vi "comm playing sender.vi"() -> ()   [LabVIEW 2009]
uses:
  UDP Lib/UDP Network Location.ctl
  <vilib>/Platform/TimedLoop/XDataNode/XDataNode.xnode
  <vilib>/Platform/TimedLoop/XDataNode/loadlvalarms.vi
  <vilib>/Platform/TimedLoop/XDataNode/timing_clust.ctl
  <vilib>/Platform/TimedLoop/XDataNode/nitl_modes.ctl
  <vilib>/Platform/TimedLoop/XDataNode/wakeup.ctl
  <vilib>/Platform/TimedLoop/XDataNode/XDNodeRunTimeDep.lvlib
panel:
  out "Network Location":T1
  out "Receive Data":string
  in  "Read Timeout":i32=1000
  in  "Local Port":u16=8800
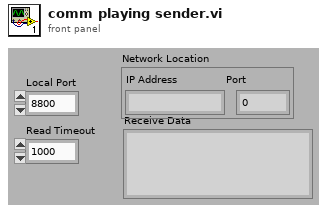
[diagram p1: front panel]
types:
  T1 = typedef "UDP Network Location.ctl" = cluster{"IP Address":string, "Port":u16}
  T2 = typedef "XDNodeRunTimeDep.lvlib/timing_clust.ctl" = cluster{"Expected End [f-1]":u64, "Actual End [f-1]":u64, "Finished Late? [f-1]":bool, "Expected End [i-1]":u64, "Actual End [i-1]":u64, "Finished Late? [i-1]":bool, "Expected Start [i]":u64, "Actual Start [i]":u64, "Expected Start [f]":u64, "Actual Start [f]":u64, "Source Name":string, "Structure Name":string, "Period":i64, "Deadline":i64, "Offset":i64, "Start":i64, "Priority":i32, "Timeout":i32, "Mode":T3, "Wakeup Reason":T4, "Error":errorcluster, "Source Type":string, "Secondary Source Type":string, "Global End Time":u64, "Global Start Time":u64, "Frame Duration":u64, "Iteration Duration":u64, "Assigned CPU":i32, "I/O Scan Engine Mode":u32}
  T3 = typedef "XDNodeRunTimeDep.lvlib/nitl_modes.ctl" = enum32{"No Change", "Process missed periods, maintain original phase", "Discard missed periods, maintain original phase", "Process missed periods, ignore original phase", "Discard missed periods, ignore original phase"}
  T4 = typedef "XDNodeRunTimeDep.lvlib/wakeup.ctl" = enum32{"Normal", "Aborted", "Asynchronous wakeup", "Timing source error", "Timed loop error", "Timeout"}
  T5 = typedef "UDP Base.ctl" = cluster{"UDP Session":refnum<k16>, "UDP Socket Params":T6}
  T6 = typedef "UDP Socket Params.ctl" = cluster{"Local Port":u16, "Read Timeout":i32, "Write Timeout":i32}
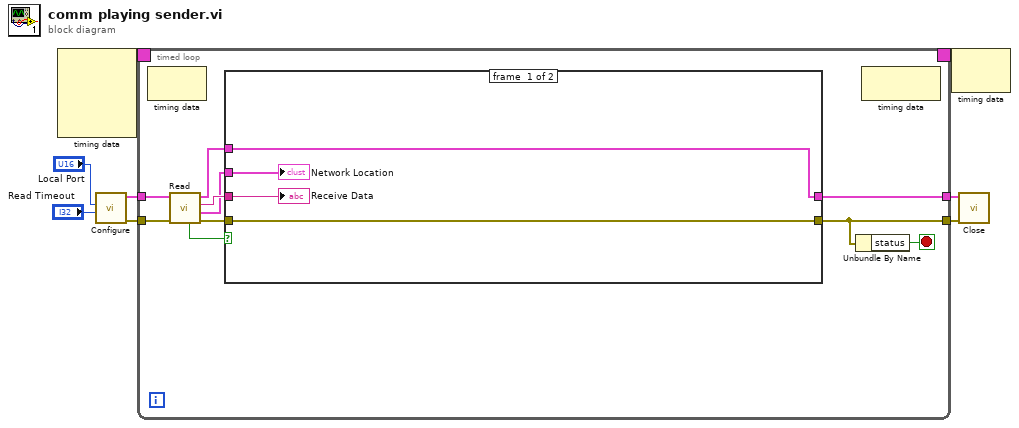
[diagram p0: block diagram]
diagram:
  n1 = node-c288() -> (w8:T2)  [unwired: 4 in]
  n2 = call "Configure.vi"("Read Timeout"="Read Timeout", "Local Port"="Local Port") -> ("error out"=w5:errorcluster, "UDP Base out"=w6:T5)  [unwired: 8 in]
  n3 = timed-loop {
    tunnel: w6 -> [w16]
    tunnel: w5 -> [w15]
    tunnel: [w18] -> w3
    tunnel: [w17] -> w4
    timing: w8 -> [_]
    timing-out: [_] -> w7
    stop <- w9 stop-if-true
    n4 = node-c288() -> ()  [unwired: 1 in, 1 out]
    n5 = call "Read.vi"("error in (no error)"=w15, "UDP Base in"=w16) -> ("error out"=w13:errorcluster, "Network Location"=w10:T1, "Receive Data"=w12:string, "UDP Base out"=w14:T5, "Timeout"=w11:bool)  [unwired: 4 in, 1 out]
    n6 = case shown="False" w11 {
      tunnel: [w21 w25] -> w18
      tunnel: [w23 w26] -> w17
      tunnel: w14 -> [w23 w26]
      tunnel: w13 -> [w21 w25]
      tunnel: w12 -> [w24 _]
      tunnel: w10 -> [w22 _]
      frame #0 {
        "Network Location" <- w22
        "Receive Data" <- w24
      }
      frame #1 {
      }
    }
    n7 = Unbundle By Name(w18) -> ("status"=w9:bool)
    n8 = node-c288() -> ()  [unwired: 1 in, 1 out]
  }
  n9 = node-c288(w7) -> ()  [unwired: 1 out]
  n10 = call "Close.vi"("error in (no error)"=w3, "Cluster of class private data"=w4) -> ()  [unwired: 9 in, 1 out]
